vi "DSF.Engine.Transceiver.Rx.vi"(8 "error in (no error)":errorcluster, 10 "Transfer Group in":refnum<class "DSF.Engine.Transfer Group.lvclass">, 11 "GE Reflective Memory Transceiver in":refnum<class "DSF.Transceiver.GE Reflective Memory.lvclass">) -> (0 "error out":errorcluster, 2 "Transfer Group out":refnum<class "DSF.Engine.Transfer Group.lvclass">, 3 "GE Reflective Memory Transceiver out":refnum<class "DSF.Transceiver.GE Reflective Memory.lvclass">)   [LabVIEW 2017, in "DSF.Transceiver.GE Reflective Memory.lvlib" / "DSF.Transceiver.GE Reflective Memory.lvclass"]
uses:
  DSF.Transceiver.GE Reflective Memory.lvclass
  Engine/Classes/Transfer/DSF.Engine.Transfer Group.lvclass
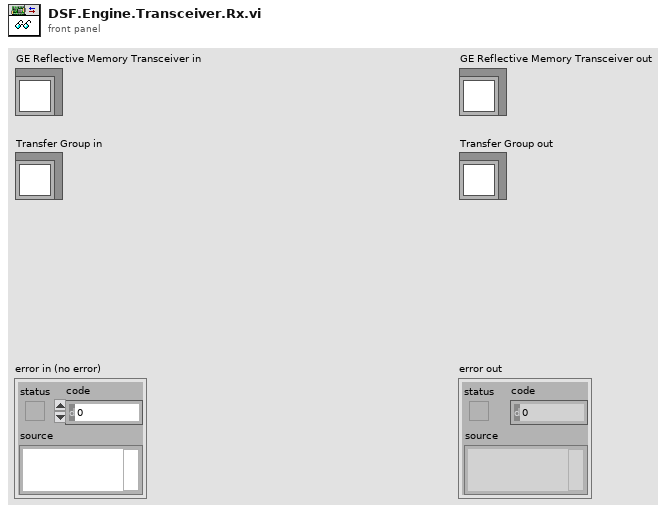
[diagram p1: front panel]
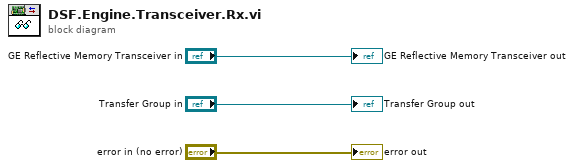
[diagram p0: block diagram]
diagram:
  "error out" <- "error in (no error)"
  "GE Reflective Memory Transceiver out" <- "GE Reflective Memory Transceiver in"
  "Transfer Group out" <- "Transfer Group in"
